vi "lib cmdline history.vi"(7 "Action":T1, 8 "error in (no error)":errorcluster, 10 "History":string[](array[string]), 11 "Text":string) -> (0 "error out":errorcluster, 2 "History out":string[](array[string]), 3 "TID list":string)   [LabVIEW 2014]
uses:
  lib cmdline enum.ctl
panel:
  out "f":i32
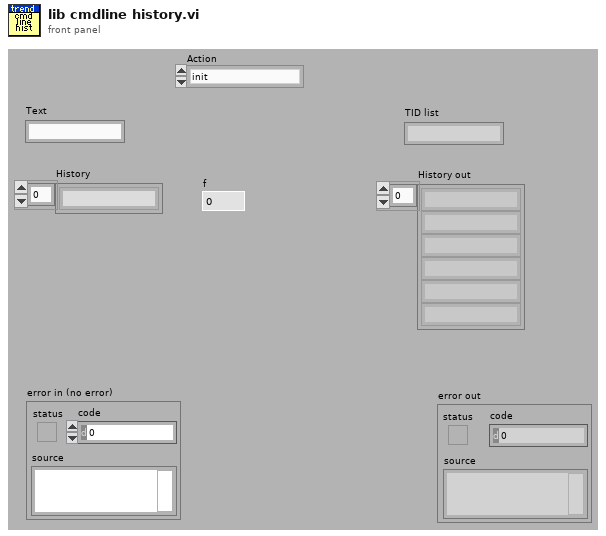
[diagram p1: front panel]
types:
  T1 = typedef "lib cmdline enum.ctl" = enum16{"init", "add", "previous", "next", "all"}
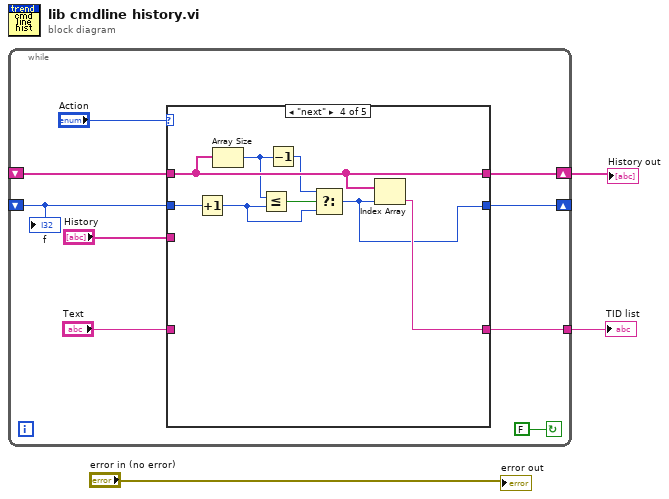
[diagram p0: block diagram]
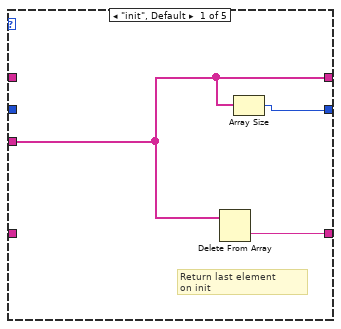
[diagram p2: hidden frame]
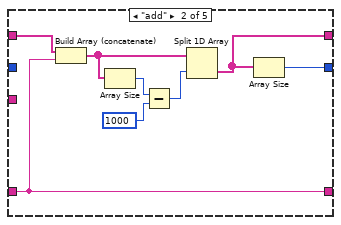
[diagram p3: hidden frame]
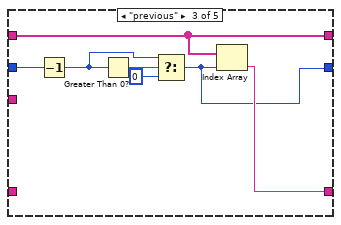
[diagram p4: hidden frame]
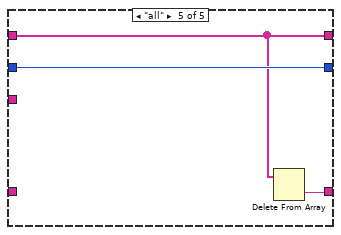
[diagram p5: hidden frame]
diagram:
  n1 = while {
    shift-right: [w10] -> w2
    shift-left: _ -> [w6]
    tunnel: [w7] -> w1
    shift-right: [w5] -> _
    shift-left: _ -> [w4]
    stop <- FALSE continue-if-true
    n2 = case shown="\"next\"" "Action" {
      tunnel: [w14 w17 w27 w34 w40] -> w10
      tunnel: "History" -> [w14 _ _ _ _]
      tunnel: "Text" -> [_ w19 _ _ _]
      tunnel: [w15 w19 w26 w36 w39] -> w7
      tunnel: w6 -> [_ w18 w27 w34 w40]
      tunnel: [w13 w16 w25 w35 w41] -> w5
      tunnel: w4 -> [_ _ w29 w37 w41]
      frame "init", Default {
        # "Return last element\non init"
        n3 = Delete From Array(array=w14) -> (deleted portion=w15:string)  [unwired: 2 in, 1 out]
        n4 = Array Size(array=w14) -> (size(s)=w13:i32)
      }
      frame "add" {
        n5 = Build Array (concatenate)(w18, w19) -> (w23:string[])
        n6 = Array Size(array=w23) -> (size(s)=w22:i32)
        n7 = Subtract(x=w22, y=1000 ("index")) -> (x-y=w20:i32)
        n8 = Split 1D Array(array=w23, index=w20) -> (second subarray=w17:string[])  [unwired: 1 out]
        n9 = Array Size(array=w17) -> (size(s)=w16:i32)
      }
      frame "previous" {
        n10 = Decrement(x=w29) -> (x-1=w24:i32)
        n11 = Greater Than 0?(x=w24) -> (x > 0?=w30:bool)
        n12 = Select(t=w24, s=w30, f=0) -> (s? t:f=w25:i32)
        n13 = Index Array(array=w27, index=w25) -> (element=w26:string)
      }
      frame "next" {
        n14 = Increment(x=w37) -> (x+1=w33:i32)
        n15 = Array Size(array=w34) -> (size(s)=w32:i32)
        n16 = Less Or Equal?(x=w32, y=w33) -> (x <= y?=w38:bool)
        n17 = Decrement(x=w32) -> (x-1=w31:i32)
        n18 = Select(t=w31, s=w38, f=w33) -> (s? t:f=w35:i32)
        n19 = Index Array(array=w34, index=w35) -> (element=w36:string)
      }
      frame "all" {
        n20 = Delete From Array(array=w40) -> (deleted portion=w39:string)  [unwired: 2 in, 1 out]
      }
    }
    "f" <- w4
  }
  "TID list" <- w1
  "History out" <- w2
  "error out" <- "error in (no error)"
